vi "Read selectedEdge.vi"(8 "error in (no error)":errorcluster, 11 "FSM.Graph in":refnum<class "FSM.Graph.lvclass">) -> (0 "error out":errorcluster, 2 "selectedEdge":i32, 3 "FSM.Graph out":refnum<class "FSM.Graph.lvclass">)   [LabVIEW 2020, in "FSM.Graph.lvclass"]
uses:
  FSM.Graph.lvclass
  FSM.Graph.lvclass/FSM.Graph.ctl
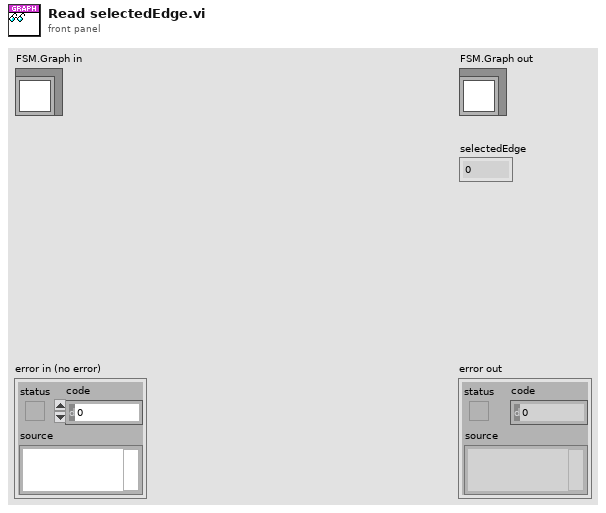
[diagram p1: front panel]
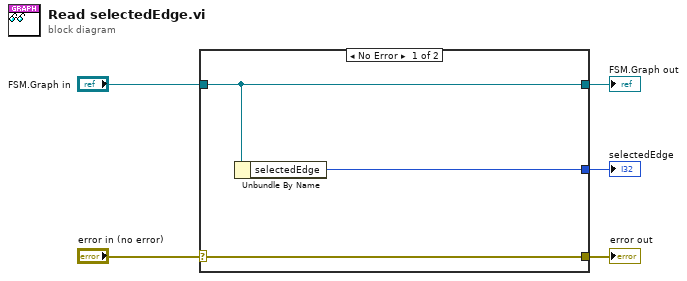
[diagram p0: block diagram]
diagram:
  n1 = case shown="No Error" "error in (no error)" {
    selector: "error in (no error)" -> [w8 w9]
    tunnel: [w8 w9] -> w4
    tunnel: [w7 w10] -> w2
    tunnel: "FSM.Graph in" -> [w7 w10]
    tunnel: [w6 _] -> w1
    frame No Error {
      n2 = Unbundle By Name(w7) -> ("selectedEdge"=w6:i32)
    }
    frame Error {
    }
  }
  "error out" <- w4
  "FSM.Graph out" <- w2
  "selectedEdge" <- w1
